vi "Store Active Controller.vi"(8 "error in (no error)":errorcluster, 10 "Controller In":refnum<class "Controller.lvclass">, 11 "Vessel in":refnum<class "Vessel.lvclass">) -> (0 "error out":errorcluster, 3 "Vessel out":refnum<class "Vessel.lvclass">)   [LabVIEW 2014, in "Vessel.lvclass"]
uses:
  Vessel.lvclass
  Controller/Controller.lvclass
  Vessel.lvclass/Vessel.ctl
  Supervisor/Supervisor.lvclass
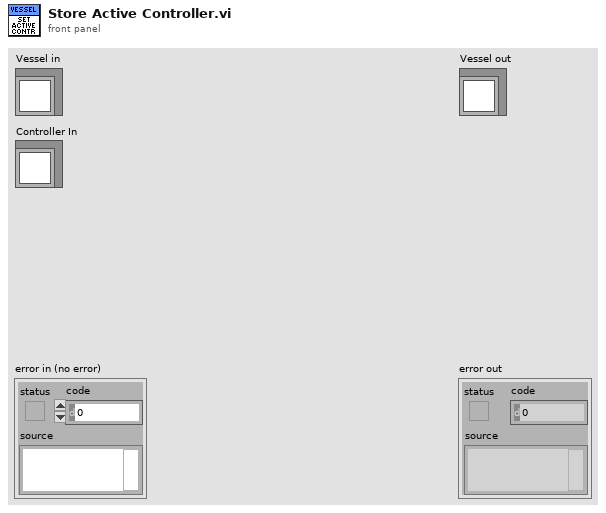
[diagram p1: front panel]
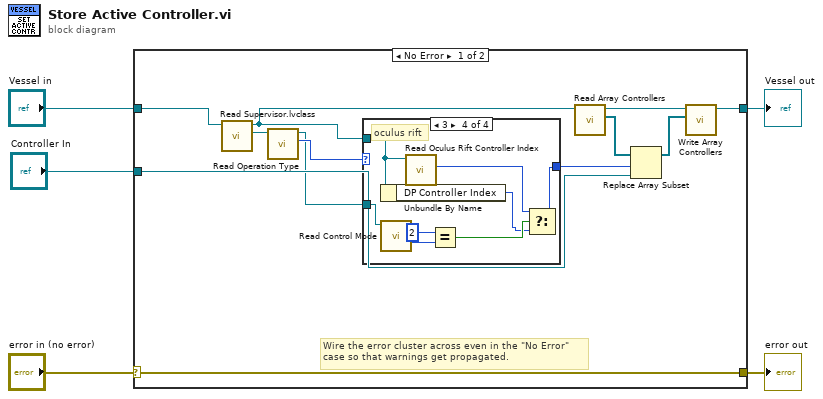
[diagram p0: block diagram]
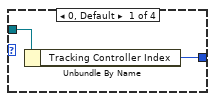
[diagram p2: hidden frame]
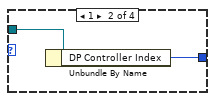
[diagram p3: hidden frame]
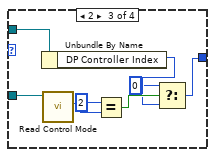
[diagram p4: hidden frame]
diagram:
  n1 = case shown="No Error" "error in (no error)" {
    selector: "error in (no error)" -> [w17 w39]
    tunnel: [w17 w39] -> w4
    tunnel: [w8 w38] -> w2
    tunnel: "Vessel in" -> [w16 w38]
    tunnel: "Controller In" -> [w13 _]
    frame No Error {
      # "Wire the error cluster across even in the \"No Error\"\ncase so that warnings get propagated."
      n2 = call "Read Supervisor.lvclass.vi"("Vessel in"=w16) -> ("Supervisor.lvclass"=w15:refnum<class "Supervisor.lvclass">, "Vessel out"=w12:refnum<class "Vessel.lvclass">)  [unwired: 8 in, 1 out]
      n3 = call-dynamic "Read Operation Type.vi"("Supervisor in"=w15) -> ("Operation Type"=w14:u16, "Supervisor out"=w7:refnum<class "Supervisor.lvclass">)  [unwired: 8 in, 1 out]
      n4 = case shown="3" w14 {
        tunnel: w12 -> [w19 w21 w29 w32]
        tunnel: [w18 w20 w23 w34] -> w6
        tunnel: w7 -> [_ _ w28 w33]
        frame 0, Default {
          n5 = Unbundle By Name(w19) -> ("Tracking Controller Index"=w18:i32)
        }
        frame 1 {
          n6 = Unbundle By Name(w21) -> ("DP Controller Index"=w20:i32)
        }
        frame 2 {
          n7 = Unbundle By Name(w29) -> ("DP Controller Index"=w24:i32)
          n8 = call-dynamic "Read Control Mode.vi"("Supervisor in"=w28) -> ("Control Mode"=w27:u16)  [unwired: 8 in, 2 out]
          n9 = Equal?(x=u16 2, y=w27) -> (x = y?=w25:bool)
          n10 = Select(t=0, s=w25, f=w24) -> (s? t:f=w23:i32)
        }
        frame 3 {
          # "oculus rift"
          n11 = Unbundle By Name(w32) -> ("DP Controller Index"=w31:i32)
          n12 = call-dynamic "Read Control Mode.vi"("Supervisor in"=w33) -> ("Control Mode"=w37:u16)  [unwired: 8 in, 2 out]
          n13 = call-dynamic "Read Oculus Rift Controller Index.vi"("Vessel in"=w32) -> ("Oculus Rift Controller Index"=w30:i32)  [unwired: 8 in, 2 out]
          n14 = Equal?(x=u16 2, y=w37) -> (x = y?=w35:bool)
          n15 = Select(t=w30, s=w35, f=w31) -> (s? t:f=w34:i32)
        }
      }
      n16 = call "Read Array Controllers.vi"("Vessel in"=w12) -> ("Array Controllers"=w10:refnum<class "Controller.lvclass">[], "Vessel out"=w11:refnum<class "Vessel.lvclass">)  [unwired: 8 in, 1 out]
      n17 = Replace Array Subset(array=w10, new element=w13, index=w6) -> (w9:refnum<class "Controller.lvclass">[])
      n18 = call "Write Array Controllers.vi"("Array Controllers"=w9, "Vessel in"=w11) -> ("Vessel out"=w8:refnum<class "Vessel.lvclass">)  [unwired: 8 in, 1 out]
    }
    frame Error {
    }
  }
  "error out" <- w4
  "Vessel out" <- w2
